vi "Verify TypeMap.vi"(6 "TypeMap in":refnum<class "TypeMap.lvclass">, 8 "error in (no error)":errorcluster, 10 "Type in":refnum<class>) -> (0 "error out":errorcluster, 2 "Type out":refnum<class>, 4 "TypeMap out":refnum<class "TypeMap.lvclass">)   [LabVIEW 2020, in "ORM_API.lvlib"]
uses:
  ORM_API.lvlib
  <vilib>/Viviota/shared/ORM.lvlibp/ORM/TypeMap/TypeMap.lvclass
  <userlib>/_OpenG.lib/lvdata/lvdata.llb/openg_variant.lvlib
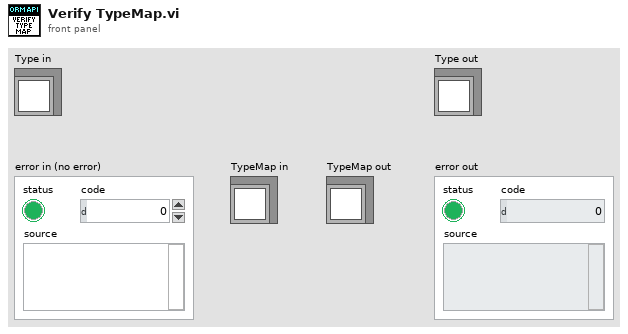
[diagram p1: front panel]
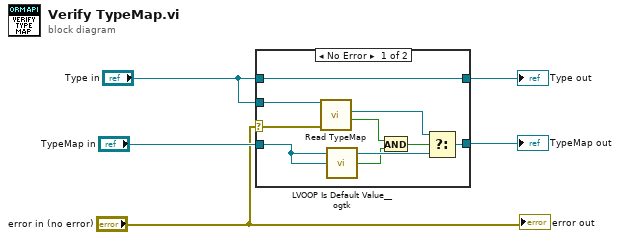
[diagram p0: block diagram]
diagram:
  n1 = case shown="No Error" "error in (no error)" {
    selector: "error in (no error)" -> [w14 _]
    tunnel: "Type in" -> [w13 _]
    tunnel: "Type in" -> [w12 w16]
    tunnel: [w12 w16] -> w2
    tunnel: "TypeMap in" -> [w9 w15]
    tunnel: [w10 w15] -> w5
    frame No Error {
      n2 = call <vilib>:"Read TypeMap.vi"("error in (no error)"=w14, "object in"=w13) -> ("found/replaced?"=w8:bool, "TypeMap in"=w11:refnum<class "TypeMap.lvclass">)  [unwired: 6 in, 2 out]
      n3 = call <userlib>:"LVOOP Is Default Value__ogtk.vi"("Object"=w9) -> ("Is Default Value?"=w7:bool)
      n4 = And(x=w8, y=w7) -> (x .and. y?=w6:bool)
      n5 = Select(t=w11, s=w6, f=w9) -> (s? t:f=w10:refnum<class "TypeMap.lvclass">)
    }
    frame Error {
    }
  }
  "TypeMap out" <- w5
  "Type out" <- w2
  "error out" <- "error in (no error)"
